vi "Pulse - Transient Off Input On.vi"(8 "error in (no error)":errorcluster, 10 "Trig Enable":bool, 11 "3300 in":refnum<class "3300.lvclass">) -> (0 "error out":errorcluster, 3 "3300 out":refnum<class "3300.lvclass">)   [LabVIEW 2019, in "3300.lvlib" / "3300.lvclass"]
uses:
  Library/3300.lvclass
  Library/3300.lvclass/3300.ctl
  Accessors/Read Local Resource.vi
  Accessors/Write Local Resource.vi
  <instrlib>/Agilent N330X Series/Agilent N330X Series.lvlib
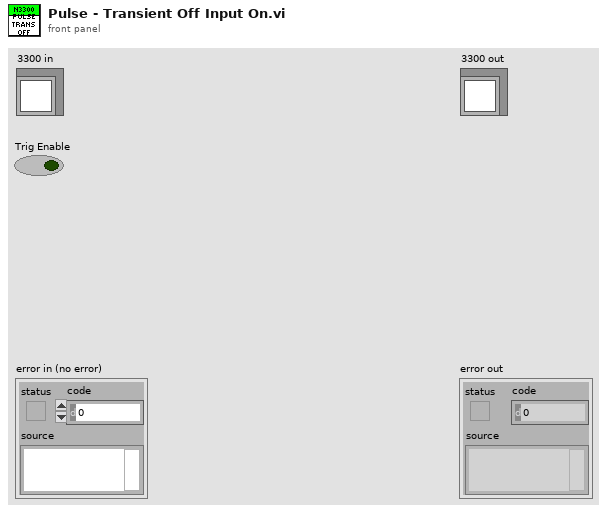
[diagram p1: front panel]
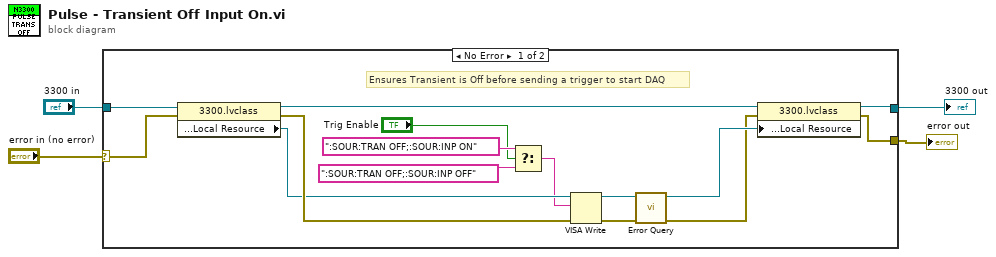
[diagram p0: block diagram]
diagram:
  n1 = case shown="No Error" "error in (no error)" {
    selector: "error in (no error)" -> [w17 w21]
    tunnel: [w11 w21] -> w1
    tunnel: [w15 w20] -> w2
    tunnel: "3300 in" -> [w9 w20]
    frame No Error {
      # "Ensures Transient is Off before sending a trigger to start DAQ"
      n2 = property class="3300.lvclass"(reference=w9, error in=w17) -> (reference out=w14:refnum<class "3300.lvclass">, error out=w16:errorcluster, "Private:Accessors:Local Resource"=w10:refnum<visa-resource-name>)
      n3 = Select(t=":SOUR:TRAN OFF;:SOUR:INP ON" ("string (\"\")"), s="Trig Enable", f=":SOUR:TRAN OFF;:SOUR:INP OFF" ("string (\"\")")) -> (s? t:f=w5:string)
      n4 = VISA Write(VISA resource name=w10, write buffer=w5, error in (no error)=w16) -> (VISA resource name out=w19:refnum<visa-resource-name>, error out=w18:errorcluster)  [unwired: 1 out]
      n5 = call <instrlib>:"Error Query.vi"("error in (no error)"=w18, "VISA resource name"=w19) -> ("error out"=w12:errorcluster, "VISA resource name out"=w13:refnum<visa-resource-name>)  [unwired: 6 in, 2 out]
      n6 = property class="3300.lvclass"(reference=w14, error in=w12, "Private:Accessors:Local Resource"=w13) -> (reference out=w15:refnum<class "3300.lvclass">, error out=w11:errorcluster)
    }
    frame Error {
    }
  }
  "error out" <- w1
  "3300 out" <- w2
